vi "Start IP Reporter.vi"(4 "ignore Gateway IP?(T)":bool=TRUE, 8 "error in (no error)":errorcluster, 10 "Init Information":string, 11 "Setttings":T1={"address"="234.5.6.7", "receiver port"=58432, "Ignore Gateway IP"=TRUE, "HostName"=""}) -> (0 "error out":errorcluster, 3 "Information Notifier":refnum<notifier>)   [LabVIEW 2017]
doc: "Starts the IP Reporter in the background and returns a notifier carrying the reported node information. Setttings carries the report address, receiver port, gateway filter and host name."
uses:
  _Typedef/Def-IniSettings -- Cluster.ctl
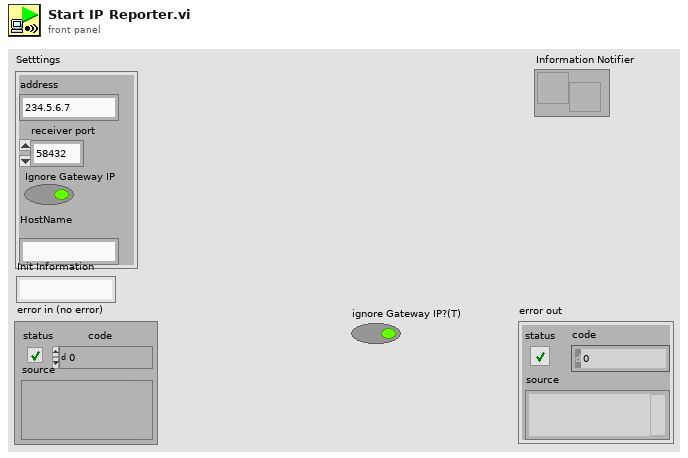
[diagram p1: front panel]
types:
  T1 = typedef "Def-IniSettings -- Cluster.ctl" = cluster{"address":string, "receiver port":u16, "Ignore Gateway IP":bool, "HostName":string}
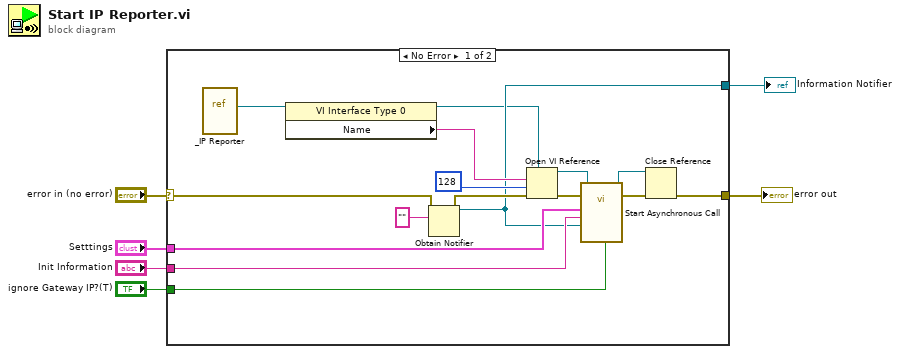
[diagram p0: block diagram]
diagram:
  n1 = case shown="No Error" "error in (no error)" {
    selector: "error in (no error)" -> [w22 w23]
    tunnel: [w16 w23] -> w5
    tunnel: "Setttings" -> [w11 _]
    tunnel: "ignore Gateway IP?(T)" -> [w10 _]
    tunnel: "Init Information" -> [w9 _]
    tunnel: [w8 _] -> w1
    frame No Error {
      n2 = vi-ref "_IP Reporter.vi"() -> (w20:refnum<vi>)
      n3 = property class="VI Interface Type 0"(reference=w20) -> (reference out=w7:refnum<vi>, "Name"=w19:string)  [unwired: 1 in, 1 out]
      n4 = Obtain Notifier(notification data type="", error in (no error)=w22) -> (notifier out=w8:refnum<notifier>, error out=w13:errorcluster)  [unwired: 2 in, 1 out]
      n5 = Open VI Reference(type specifier VI Refnum (for type only)=w7, vi path=w19, options=128, error in (no error)=w13) -> (vi reference=w14:refnum<vi>, error out=w21:errorcluster)  [unwired: 2 in]
      n6 = call-by-ref "Start Asynchronous Call"(reference=w14, error in=w21, "ignore Gateway IP?(T)"=w10, "notifier"=w8, "Init-Information"=w9, "Setttings"=w11) -> (reference out=w15:refnum<vi>, error out=w17:errorcluster)  [unwired: 7 in, 1 out]
      n7 = Close Reference(reference=w15, error in (no error)=w17) -> (error out=w16:errorcluster)
    }
    frame Error {
    }
  }
  "error out" <- w5
  "Information Notifier" <- w1
